vi "Framework Test.vi"() -> ()   [LabVIEW 2017]
uses:
  Typedefs/DSF Engine Framework Configuration.ctl
  Typedefs/DSF Engine Plugin Configuration.ctl
  Typedefs/Core Plugin Configuration.ctl
  Typedefs/DSF Timing Info.ctl
  Typedefs/DSF Settings Info.ctl
  Typedefs/DSF Engine Plugin Thread Configuration.ctl
  Typedefs/Core Thread Configuration.ctl
  Typedefs/DSF Engine Transfer Group Configuration.ctl
  Typedefs/Core Group Configuration.ctl
  Typedefs/DSF Direction.ctl
  Typedefs/DSF Timeout Behavior.ctl
  Typedefs/DSF Engine Transfer Configuration.ctl
  Typedefs/Core Transfer Configuration.ctl
  Typedefs/DSF Engine Channel Configuration.ctl
  Typedefs/Core Channel Configuration.ctl
  Typedefs/DSF Data Type.ctl
  Classes/Framework/Framework Options.ctl
  Typedefs/DSF FIFO Options.ctl
  Classes/Thread/Thread Options.ctl
  Typedefs/DSF Plugin Options.ctl
  Typedefs/DSF Performance Options.ctl
  Classes/Framework/Data Server Options.ctl
  Classes/Configuration/Core/Core Configuration.lvclass/Core Configuration.ctl
  Classes/Configuration/Core/Transfer/Transfer Configuration.lvclass/Transfer Configuration.ctl
  Classes/Configuration/Core/Group/Group Configuration.lvclass/Group Configuration.ctl
  Classes/Configuration/Core/Thread/Thread Configuration.lvclass/Thread Configuration.ctl
  Classes/Configuration/Core/Plugin/Plugin Configuration.lvclass/Plugin Configuration.ctl
  Classes/Configuration/Core/Framework/Framework Configuration.lvclass/Framework Configuration.ctl
  <vilib>/NI/Memory Manager/Classes/Pointer/Pointer.lvclass/Pointer.ctl
  Classes/Framework/Framework.lvclass/Framework.ctl
  <vilib>/NI/Memory Manager/Classes/Pointer/Write Bool.vi
  <vilib>/NI/Memory Manager/Classes/Pointer/Write DBL.vi
  <vilib>/NI/Memory Manager/Classes/Pointer/Read Bool.vi
  <vilib>/NI/Memory Manager/Classes/Pointer/Set Address.vi
  <vilib>/NI/Memory Manager/Classes/Pointer/Set Size.vi
  <vilib>/NI/Memory Manager/Classes/Pointer/Set Internal.vi
  <vilib>/NI/Memory Manager/Classes/Pointer/Check Null Pointer.vi
  <vilib>/NI/Memory Manager/Classes/Pointer/Clear (No Check).vi
  <vilib>/NI/Memory Manager/Classes/Pointer/Check Length.vi
  <vilib>/NI/Memory Manager/Classes/Pointer/Write (No Check).vi
  <vilib>/NI/Memory Manager/Classes/Pointer/Write (No Check) Bool.vi
  <vilib>/NI/Memory Manager/Classes/Pointer/Check Move.vi
  <vilib>/NI/Memory Manager/Classes/Pointer/Write (No Check) DBL.vi
  <vilib>/NI/Memory Manager/Classes/Pointer/Read (No Check).vi
  <vilib>/NI/Memory Manager/Classes/Pointer/Read (No Check) Bool.vi
  <vilib>/NI/Memory Manager/Classes/Pointer/Get Internal.vi
  <vilib>/NI/Memory Manager/Classes/Pointer/Errors.vi
  <vilib>/NI/Memory Manager/Classes/Pointer/Zone.vi
  Classes/Configuration/Core/Set Component Settings.vi
  <vilib>/NI/Memory Manager/Classes/Pointer/Null Pointer.vi
  <vilib>/NI/Memory Manager/Classes/Pointer/Is Null.vi
  <vilib>/NI/Memory Manager/Classes/Pointer/Check Bounds (Pointer).vi
  <vilib>/NI/Memory Manager/Classes/Pointer/Check Count.vi
  <vilib>/NI/Memory Manager/Classes/Pointer/Check Bounds (Power of 2).vi
  <vilib>/NI/Memory Manager/Classes/Pointer/Create Error.vi
  <vilib>/NI/Memory Manager/Classes/Pointer/Out of Bounds.vi
  <vilib>/NI/Memory Manager/Classes/Pointer/Check Bounds.vi
  <vilib>/NI/Memory Manager/Constants/Constants.vi
  <vilib>/NI/Memory Manager/Constants/Library Name.vi
  <vilib>/NI/Memory Manager/Classes/Pointer/Pointer Error Info.vi
  <vilib>/NI/Memory Manager/Constants/Pointer Class Name.vi
  <vilib>/NI/Memory Manager/Classes/Pointer/Write Pointer Size to Error.vi
  <vilib>/NI/Memory Manager/Classes/Pointer/Check Bounds (Buffer).vi
  <vilib>/NI/Memory Manager/Classes/Pointer/Buffer Underflow.vi
  Classes/Configuration/Core/Plugin/Plugin Configuration.lvclass
  C:/Git/niveristand-data-sharing-framework-custom-device/Core/Classes/Configuration/Core/Core Configuration.lvclass
  Classes/Configuration/Core/Thread/Thread Configuration.lvclass
  Classes/Configuration/Core/Group/Group Configuration.lvclass
  Classes/Configuration/Core/Transfer/Transfer Configuration.lvclass
  <vilib>/NI/Memory Manager/VIs/New Error Cluster.vi
  <vilib>/NI/Memory Manager/VIs/New Error Cluster (512B).vi
  <vilib>/NI/Memory Manager/VIs/Set Error Status.vi
  <vilib>/NI/Memory Manager/VIs/Set Error Code.vi
  <vilib>/NI/Memory Manager/VIs/Set Error Source.vi
  <vilib>/NI/Memory Manager/VIs/Write String to Source.vi
  <vilib>/NI/Memory Manager/VIs/Write Numeric to Source.vi
  <vilib>/NI/Memory Manager/VIs/Write Numeric Scalar to Source (Base10 U64).vi
  Classes/Framework/Increment Plugins.vi
  Classes/Framework/Update Performance.vi
  Classes/Framework/Update Status.vi
  Classes/Configuration/Core/Framework/Framework Configuration.lvclass
  <vilib>/NI/Memory Manager/Classes/Pointer/Pointer.lvclass
  Classes/Framework/Framework.lvclass
  Classes/Configuration Session/Configuration Session.lvclass
  DSF Core.lvlib
  Classes/Thread/Thread.lvclass
  Classes/Configuration/Core/Channel/Channel Configuration.lvclass
panel:
  in  "channel index":u64
  in  "channel data":dbl format="%.3f"
  out "iteration":u64
  out "error out":errorcluster
  in  "framework options":T1={"FIFO Options"={"Infinite Timeouts"=FALSE}, "Thread Options"={"Show FP On Call"=TRUE, "Close FP After Call"=TRUE, "Allow Debugging"=TRUE}, "Plugin Options"={"Default Components"=FALSE}, "Performance Options"={"Measure Period"=TRUE, "Measure Rx/Tx Duration"=TRUE}, "Data Server Options"={"Enable Data Server"=TRUE, "Period"=50}} {"Data Server Options"."Period" format="%d ms"}
  in  "framework configuration":T7={"plugins"=[{"core"={"name"="Plugin", "components"=["Default Buffer Converter"], "cycle timing"={"priority"=10000, "decimation"=1, "offset"=0}}, "component settings"=[], "threads"=[{"core"={"processor"=-2, "priority offset"=0}, "component settings"=[], "transfer groups"=[{"core"={"name"="Group", "direction"=enum."Tx", "cycle timing"={"priority"=100, "decimation"=1, "offset"=0}, "timeout behavior"=enum."Increment Late Count", "enable conversion"=TRUE}, "component settings"=[], "transfers"=[{"core"={"name"="Transfer"}, "component settings"=[], "channels"=[{"core"={"name"="Channel", "units"="V DBL", "engine data type"=enum."DBL", "string data type"=enum."DBL", "string offset"=0}, "component settings"=[]}, {"core"={"name"="Channel", "units"="V SGL", "engine data type"=enum."DBL", "string data type"=enum."SGL", "string offset"=8}, "component settings"=[]}, {"core"={"name"="Channel", "units"="I32", "engine data type"=enum."DBL", "string data type"=enum."I32", "string offset"=12}, "component settings"=[]}, {"core"={"name"="Channel", "units"="U32", "engine data type"=enum."DBL", "string data type"=enum."U32", "string offset"=16}, "component settings"=[]}, {"core"={"name"="Channel", "units"="U64", "engine data type"=enum."DBL", "string data type"=enum."U64", "string offset"=20}, "component settings"=[]}, {"core"={"name"="Channel", "units"="Bool", "engine data type"=enum."DBL", "string data type"=enum."Bool", "string offset"=28}, "component settings"=[]}, {"core"={"name"="Channel", "units"="U8", "engine data type"=enum."DBL", "string data type"=enum."U8", "string offset"=29}, "component settings"=[]}]}]}]}]}]}
  in  "stop":bool
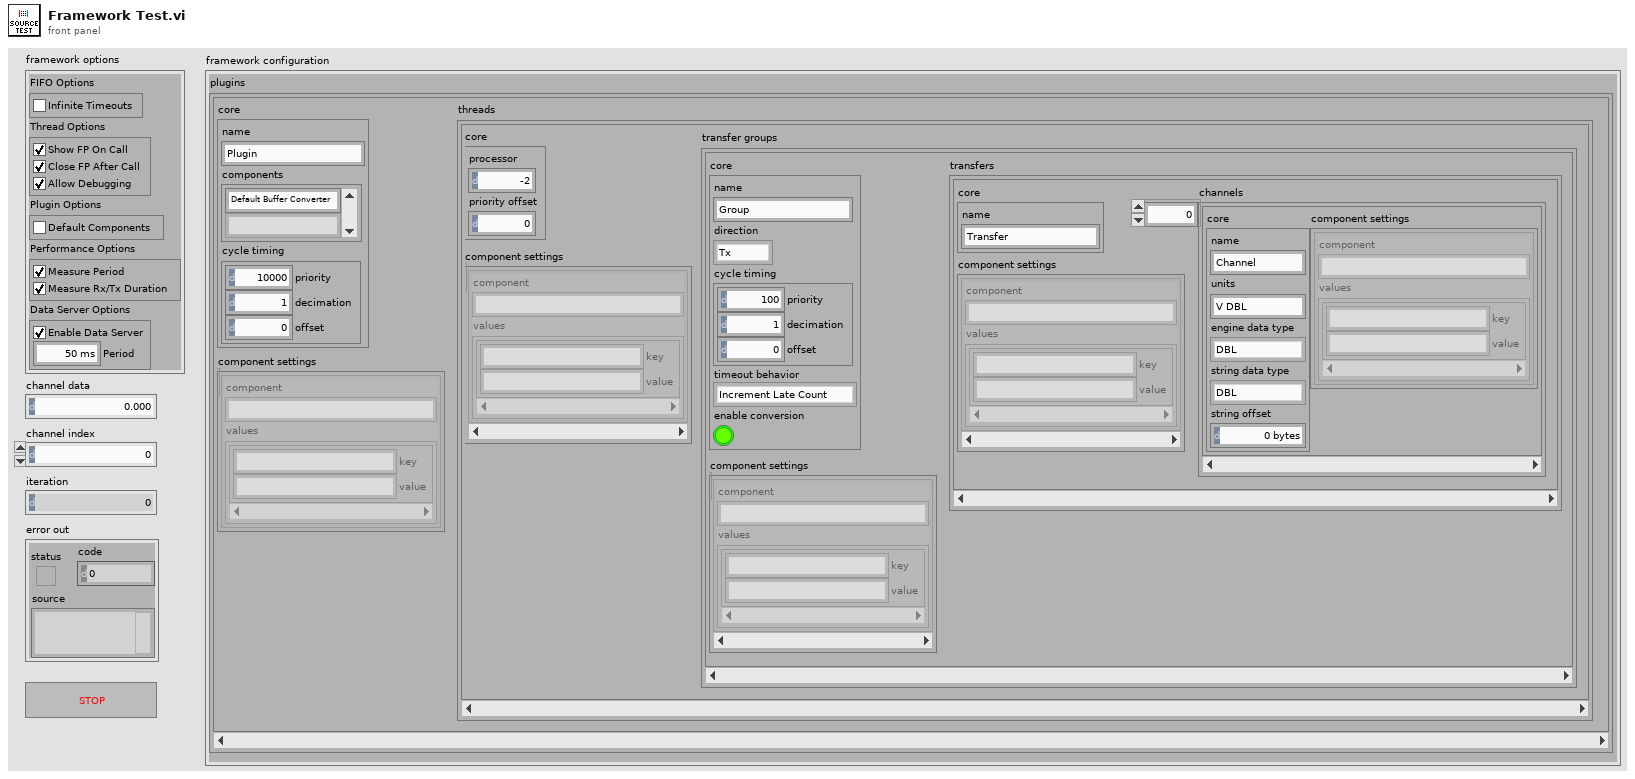
[diagram p1: front panel]
types:
  T1 = typedef "DSF Core.lvlib/Framework.lvclass/Framework Options.ctl" = cluster{"FIFO Options":T2, "Thread Options":T3, "Plugin Options":T4, "Performance Options":T5, "Data Server Options":T6}
  T2 = typedef "DSF Core.lvlib/Framework.lvclass/DSF FIFO Options.ctl" = cluster{"Infinite Timeouts":bool}
  T3 = typedef "DSF Core.lvlib/Thread.lvclass/Thread Options.ctl" = cluster{"Show FP On Call":bool, "Close FP After Call":bool, "Allow Debugging":bool}
  T4 = typedef "DSF Core.lvlib/Framework.lvclass/DSF Plugin Options.ctl" = cluster{"Default Components":bool}
  T5 = typedef "DSF Core.lvlib/DSF Performance Options.ctl" = cluster{"Measure Period":bool, "Measure Rx/Tx Duration":bool}
  T6 = typedef "DSF Core.lvlib/Framework.lvclass/Data Server Options.ctl" = cluster{"Enable Data Server":bool, "Period":u32}
  T7 = typedef "DSF Core.lvlib/DSF Engine Framework Configuration.ctl" = cluster{"plugins":T8[]}
  T8 = typedef "DSF Core.lvlib/DSF Engine Plugin Configuration.ctl" = cluster{"core":T9, "component settings":T11[], "threads":T12[]}
  T9 = typedef "DSF Core.lvlib/Plugin Configuration.lvclass/Core Plugin Configuration.ctl" = cluster{"name":string, "components":string[], "cycle timing":T10}
  T10 = typedef "DSF Core.lvlib/DSF Timing Info.ctl" = cluster{"priority":u64, "decimation":u64, "offset":u64}
  T11 = typedef "DSF Core.lvlib/DSF Settings Info.ctl" = cluster{"component":string, "values":cluster{"key":string, "value":string}[]}
  T12 = typedef "DSF Core.lvlib/DSF Engine Plugin Thread Configuration.ctl" = cluster{"core":T13, "component settings":T11[], "transfer groups":T14[]}
  T13 = typedef "DSF Core.lvlib/Thread Configuration.lvclass/Core Thread Configuration.ctl" = cluster{"processor":i32, "priority offset":i16}
  T14 = typedef "DSF Core.lvlib/DSF Engine Transfer Group Configuration.ctl" = cluster{"core":T15, "component settings":T11[], "transfers":T18[]}
  T15 = typedef "DSF Core.lvlib/Group Configuration.lvclass/Core Group Configuration.ctl" = cluster{"name":string, "direction":T16, "cycle timing":T10, "timeout behavior":T17, "enable conversion":bool}
  T16 = typedef "DSF Core.lvlib/DSF Direction.ctl" = enum8{"Tx", "Rx"}
  T17 = typedef "DSF Core.lvlib/DSF Timeout Behavior.ctl" = enum8{"Increment Late Count", "Throw Error"}
  T18 = typedef "DSF Core.lvlib/DSF Engine Transfer Configuration.ctl" = cluster{"core":T19, "component settings":T11[], "channels":T20[]}
  T19 = typedef "DSF Core.lvlib/Transfer Configuration.lvclass/Core Transfer Configuration.ctl" = cluster{"name":string}
  T20 = typedef "DSF Core.lvlib/DSF Engine Channel Configuration.ctl" = cluster{"core":T21, "component settings":T11[]}
  T21 = typedef "DSF Core.lvlib/Channel Configuration.lvclass/Core Channel Configuration.ctl" = cluster{"name":string, "units":string, "engine data type":T22, "string data type":T22, "string offset":u64}
  T22 = typedef "DSF Core.lvlib/DSF Data Type.ctl" = enum8{"Bool", "SGL", "DBL", "I8", "I16", "I32", "I64", "U8", "U16", "U32", "U64"}
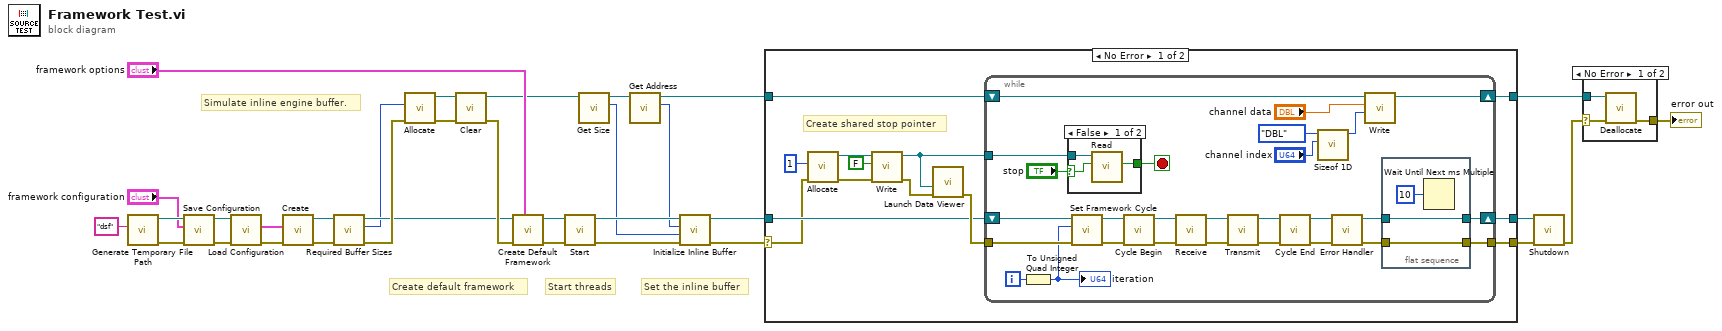
[diagram p0: block diagram]
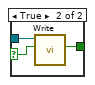
[diagram p3: hidden frame]
diagram:
  # "Set the inline buffer"
  # "Start threads"
  # "Create default framework"
  # "Simulate inline engine buffer."
  n1 = call <vilib>:"Generate Temporary File Path.vi"("Temporary File Extension (tmp)"="dsf") -> ("error out"=w16:errorcluster, "Unique Temporary File Path"=w19:path)  [unwired: 9 in]
  n2 = call "Save Configuration.vi"("error in (no error)"=w16, "framework configuration"="framework configuration", "configuration file path"=w19) -> ("error out"=w18:errorcluster, "configuration file path dup"=w17:path)  [unwired: 5 in, 2 out]
  n3 = call "Load Configuration.vi"("error in (no error)"=w18, "configuration file path"=w17) -> ("error out"=w10:errorcluster, "framework configuration"=w9:T7)  [unwired: 6 in, 2 out]
  n4 = call "Create.vi"("error in (no error)"=w10, "framework configuration"=w9) -> ("error out"=w7:errorcluster, "Framework Configuration out"=w8:refnum<class "Framework Configuration.lvclass">)  [unwired: 8 in]
  n5 = call-dynamic "Required Buffer Sizes.vi"("error in (no error)"=w7, "Framework Configuration in"=w8) -> ("error out"=w15:errorcluster, "engine size"=w12:u64, "Framework Configuration out"=w14:refnum<class "Framework Configuration.lvclass">)  [unwired: 6 in, 1 out]
  n6 = call <vilib>:"Allocate.vi"("error in (no error)"=w15, "size"=w12) -> ("error out"=w29:errorcluster, "Pointer out"=w26:refnum<class "Pointer.lvclass">)  [unwired: 8 in]
  n7 = call <vilib>:"Clear.vi"("error in (no error)"=w29, "Pointer in"=w26) -> ("error out"=w33:errorcluster, "Pointer out"=w5:refnum<class "Pointer.lvclass">)  [unwired: 8 in]
  n8 = call "Create Default Framework.vi"("framework options"="framework options", "error in (no error)"=w33, "Framework Configuration"=w14) -> ("error out"=w23:errorcluster, "Framework"=w25:refnum<class "Framework.lvclass">)  [unwired: 7 in]
  n9 = call-dynamic "Start.vi"("error in (no error)"=w23, "Framework in"=w25) -> ("error out"=w24:errorcluster, "Framework out"=w32:refnum<class "Framework.lvclass">)  [unwired: 8 in]
  n10 = call <vilib>:"Get Size.vi"("Pointer in"=w5) -> ("size"=w28:u64, "Pointer out"=w6:refnum<class "Pointer.lvclass">)  [unwired: 9 in]
  n11 = call <vilib>:"Get Address.vi"("Pointer in"=w6) -> ("address"=w27:u64, "Pointer out"=w4:refnum<class "Pointer.lvclass">)  [unwired: 9 in]
  n12 = call "Initialize Inline Buffer.vi"("error in (no error)"=w24, "size"=w28, "address"=w27, "Framework in"=w32) -> ("error out"=w22:errorcluster, "Framework out"=w21:refnum<class "Framework.lvclass">)  [unwired: 6 in]
  n13 = case shown="No Error" w22 {
    selector: w22 -> [w35 w84]
    tunnel: [w45 w84] -> w31
    tunnel: w21 -> [w42 w85]
    tunnel: [w46 w85] -> w30
    tunnel: w4 -> [w44 w83]
    tunnel: [w41 w83] -> w3
    frame No Error {
      # "Create shared stop pointer"
      n14 = call <vilib>:"Allocate.vi"("error in (no error)"=w35, "size"=u64 1) -> ("error out"=w36:errorcluster, "Pointer out"=w40:refnum<class "Pointer.lvclass">)  [unwired: 8 in]
      n15 = call-poly <vilib>:"Write.vi"("error in (no error)"=w36, "value"=FALSE, "Pointer in"=w40) -> ("error out"=w34:errorcluster, "Pointer out"=w38:refnum<class "Pointer.lvclass">)  [unwired: 5 in, 2 out]
      n16 = call "Launch Data Viewer.vi"("error in (no error)"=w34, "stop pointer"=w38) -> ("error out"=w43:errorcluster)  [unwired: 9 in]
      n17 = while {
        shift-right: [w71] -> w46
        shift-left: w42 -> [w65]
        tunnel: w38 -> [w68]
        tunnel: w43 -> [w64]
        tunnel: [w70] -> w45
        shift-right: [w47] -> w41
        shift-left: w44 -> [w52]
        i -> [w69]
        stop <- w66 stop-if-true
        n18 = To Unsigned Quad Integer(1:w69) -> (0:w63:u64)
        "iteration" <- w63
        n19 = case shown="False" "stop" {
          selector: "stop" -> [w75 w78]
          tunnel: w68 -> [w76 w79]
          tunnel: [w74 w77] -> w66
          frame False {
            n20 = call-poly <vilib>:"Read.vi"("value in"=w75, "Pointer in"=w76) -> ("value out"=w74:bool)  [unwired: 6 in, 3 out]
          }
          frame True {
            n21 = call-poly <vilib>:"Write.vi"("value"=w78, "Pointer in"=w79) -> ("value"=w77:bool)  [unwired: 6 in, 3 out]
          }
        }
        n22 = call "Set Framework Cycle.vi"("error in (no error)"=w64, "iteration"=w63, "Framework in"=w65) -> ("error out"=w61:errorcluster, "Framework out"=w62:refnum<class "Framework.lvclass">)  [unwired: 7 in]
        n23 = call "Cycle Begin.vi"("error in (no error)"=w61, "Framework in"=w62) -> ("error out"=w59:errorcluster, "Framework out"=w60:refnum<class "Framework.lvclass">)  [unwired: 8 in]
        n24 = call "Receive.vi"("error in"=w59, "framework in"=w60) -> ("error out"=w73:errorcluster, "framework out"=w72:refnum<class "Framework.lvclass">)  [unwired: 8 in]
        n25 = call "Transmit.vi"("error in"=w73, "framework in"=w72) -> ("error out"=w57:errorcluster, "framework out"=w58:refnum<class "Framework.lvclass">)  [unwired: 8 in]
        n26 = call "Cycle End.vi"("error in (no error)"=w57, "Framework in"=w58) -> ("error out"=w55:errorcluster, "Framework out"=w56:refnum<class "Framework.lvclass">)  [unwired: 8 in]
        n27 = call "Sizeof 1D.vi"("count"="channel index", "data type"=DSF_Data_Type."DBL") -> ("size in bytes"=w48:u64)  [unwired: 9 in]
        n28 = call "Error Handler.vi"("error in (no error)"=w55, "Framework in"=w56) -> ("error out"=w53:errorcluster, "Framework out"=w54:refnum<class "Framework.lvclass">)  [unwired: 8 in]
        n29 = call-poly <vilib>:"Write.vi"("offset (0)"=w48, "value"="channel data", "Pointer in"=w52) -> ("Pointer out"=w47:refnum<class "Pointer.lvclass">)  [unwired: 5 in, 3 out]
        n30 = flat-sequence {
          tunnel: w54 -> [w81]
          tunnel: w53 -> [w80]
          tunnel: [w81] -> w71
          tunnel: [w80] -> w70
          frame #0 {
            n31 = Wait Until Next ms Multiple(millisecond multiple=u32 10 ("milliseconds to wait")) -> ()  [unwired: 1 out]
          }
        }
      }
    }
    frame Error {
    }
  }
  n32 = call-dynamic "Shutdown.vi"("error in (no error)"=w31, "Framework in"=w30) -> ("error out"=w2:errorcluster)  [unwired: 8 in, 1 out]
  n33 = case shown="No Error" w2 {
    selector: w2 -> [w87 w89]
    tunnel: w3 -> [w88 _]
    tunnel: [w86 w89] -> w1
    frame No Error {
      n34 = call <vilib>:"Deallocate.vi"("error in (no error)"=w87, "Pointer"=w88) -> ("error out"=w86:errorcluster)  [unwired: 8 in, 1 out]
    }
    frame Error {
    }
  }
  "error out" <- w1
